vi "DHE_DRV_expose.vi"(0 "fd":i32, 1 "num_prevex":i32, 2 "num_postex":i32, 5 "bytes_to_receive":i32, 7 "fast":bool, 9 "expt_time":u32, 11 "error in (no error)":errorcluster, 12 "num_coadds":i32, 13 "npics":i32, 14 "num_sur":i32) -> (4 "fd out":i32, 6 "bytes_to_receive":i32, 8 "num_prevex out":u32, 10 "return value":i32, 15 "error out":errorcluster)   [LabVIEW 2016]
doc: "This VI closes the I/O interface with the instrument."
uses:
  c/lib/libarcDHE.so
panel:
  out "num_postex out":u32
  out "expt_time":u32
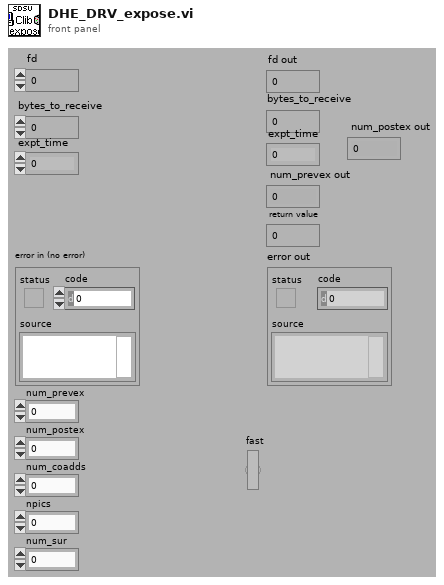
[diagram p1: front panel]
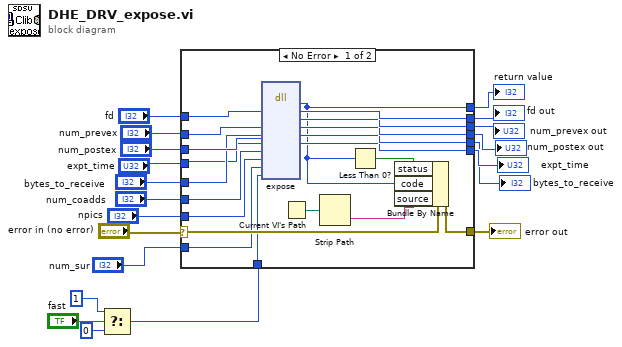
[diagram p0: block diagram]
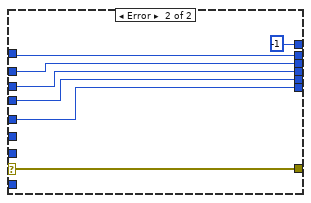
[diagram p2: hidden frame]
diagram:
  n1 = Select(t=1, s="fast", f=0) -> (s? t:f=w1:i32)
  n2 = case shown="No Error" "error in (no error)" {
    selector: "error in (no error)" -> [w36 w46]
    tunnel: [w27 -1] -> w20
    tunnel: [w37 w46] -> w19
    tunnel: "fd" -> [w33 w45]
    tunnel: "num_prevex" -> [w34 w44]
    tunnel: "expt_time" -> [w25 w42]
    tunnel: "bytes_to_receive" -> [w26 w41]
    tunnel: "num_postex" -> [w35 w43]
    tunnel: [w32 w45] -> w12
    tunnel: [w31 w44] -> w11
    tunnel: [w30 w43] -> w10
    tunnel: [w29 w42] -> w8
    tunnel: [w28 w41] -> w9
    tunnel: "num_coadds" -> [w24 _]
    tunnel: "npics" -> [w23 _]
    tunnel: "num_sur" -> [w22 _]
    tunnel: w1 -> [w21 _]
    frame No Error {
      n3 = dll-call lib="home/simager/panview/PAN/Modules/SDSU/private/c/lib/libarcDHE.so" fn="expose"("fd"=w33, "num_prevex"=w34, "num_postex"=w35, "bytes_per_image"=w26, "exp_time"=w25, "num_coadds"=w24, "npics"=w23, "num_sur"=w22, "fast"=w21) -> ("return type"=w27:i32, "fd"=w32:i32, "num_prevex"=w31:i32, "num_postex"=w30:i32, "bytes_per_image"=w29:i32, "exp_time"=w28:i32)  [unwired: 7 in, 2 out]
      n4 = Current VI's Path() -> (path=w39:path)
      n5 = Strip Path(path=w39) -> (name=w38:string)  [unwired: 1 out]
      n6 = Less Than 0?(x=w27) -> (x < 0?=w40:bool)
      n7 = Bundle By Name(cluster=w36, "status"=w40, "code"=w27, "source"=w38) -> (w37:errorcluster)
    }
    frame Error {
    }
  }
  "error out" <- w19
  "return value" <- w20
  "bytes_to_receive" <- w8
  "num_prevex out" <- w11
  "fd out" <- w12
  "expt_time" <- w9
  "num_postex out" <- w10
